vi "whilexample.vi"() -> ()   [LabVIEW 2015]
panel:
  in  "stop":bool
  out "Mensaje de\n control:":string
  out "Advertencia":bool
  in  "Temperatura minima\npermitida":dbl
  in  "Temperatura Maxima\npermitida":dbl
  in  "Temperatura (F)":dbl
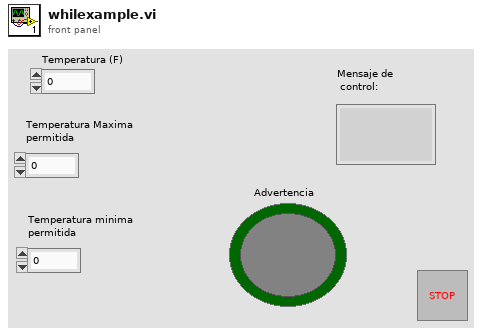
[diagram p1: front panel]
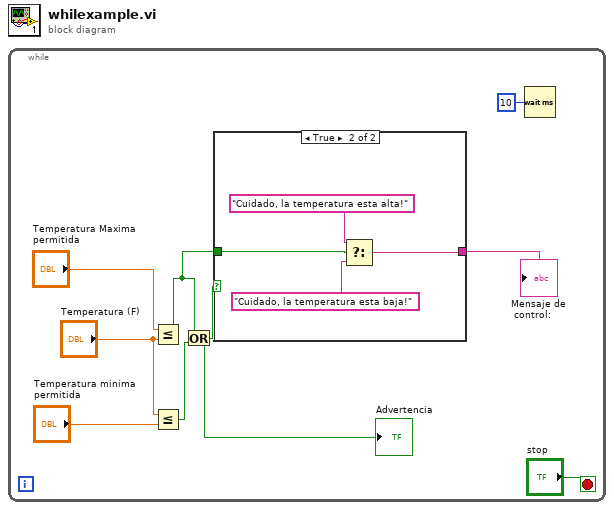
[diagram p0: block diagram]
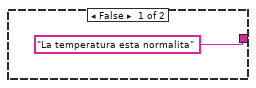
[diagram p2: hidden frame]
diagram:
  n1 = while {
    stop <- "stop" stop-if-true
    n2 = Less Or Equal?(x="Temperatura Maxima\npermitida", y="Temperatura (F)") -> (x <= y?=w4:bool)
    n3 = Less Or Equal?(x="Temperatura (F)", y="Temperatura minima\npermitida") -> (x <= y?=w6:bool)
    n4 = Or(x=w4, y=w6) -> (x .or. y?=w5:bool)
    "Advertencia" <- w5
    n5 = case shown="True" w5 {
      tunnel: w4 -> [_ w14]
      tunnel: ["La temperatura esta normalita" w11] -> w3
      frame False {
      }
      frame True {
        n6 = Select(t="Cuidado, la temperatura esta alta!", s=w14, f="Cuidado, la temperatura esta baja!") -> (s? t:f=w11:string)
      }
    }
    "Mensaje de\n control:" <- w3
    n7 = Wait (ms)(milliseconds to wait=u32 10) -> ()  [unwired: 1 out]
  }
